vi "StopRequest.vi"(8 "error in (no error)":errorcluster, 9 "Wait for Module to stop? (F)":bool, 11 "ModuleAdmin":refnum<class "ModuleAdmin.lvclass">) -> (0 "error out":errorcluster, 2 "Stop Request Sent":bool)   [LabVIEW 2017, in "PmuImpairModule.lvlib"]
uses:
  PmuImpairModule.lvlib
  <userlib>/NIST/ModuleAdminLib/ModuleAdmin/ModuleAdmin.lvclass
  <vilib>/event_ctls.llb/usereventprio.ctl
  PublicAPI/Arguments/Requests/clStopArgument.ctl
  clEventType.ctl
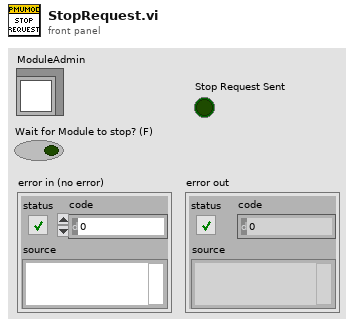
[diagram p1: front panel]
types:
  T1 = typedef "PmuImpairModule.lvlib/clRequestEvents.ctl" = cluster{"StopRequest":refnum<user-event>, "LoadPluginRequest":refnum<user-event>, "WriteImpairConfig":refnum<user-event>, "ReadImpairConfig":refnum<user-event>, "WriteImpairParams":refnum<user-event>, "ReadImpairParams":refnum<user-event>, "WriteEvtReports":refnum<user-event>, "GetImpairReports":refnum<user-event>, "ReadPathToPluginRequest":refnum<user-event>, "WriteEvtSignal":refnum<user-event>, "WriteEvtConfig":refnum<user-event>, "WriteEvtParams":refnum<user-event>, "ReadBusNumber":refnum<user-event>, "WriteBusNumber":refnum<user-event>, "ShowPanel":refnum<user-event>}
  T2 = typedef "PmuImpairModule.lvlib/clEventType.ctl" = cluster{"ModuleID":i32, "Data":variant}
  T3 = typedef "PmuImpairModule.lvlib/clStopArgument.ctl" = cluster{"Exit via Stop Module Req?":bool, "Wait for Module to stop?":bool, "ModuleAdmin":refnum<class "ModuleAdmin.lvclass">}
  T4 = typedef "usereventprio.ctl" = enum32{"high priority", "normal priority"}
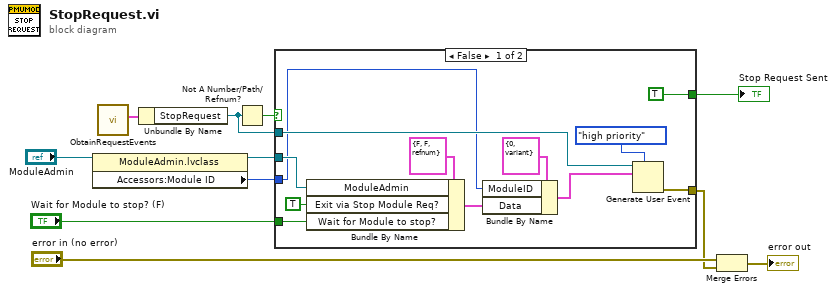
[diagram p0: block diagram]
diagram:
  n1 = property class="ModuleAdmin.lvclass"(reference="ModuleAdmin") -> (reference out=w2:refnum<class "ModuleAdmin.lvclass">, "Accessors:Module ID"=w1:i32)  [unwired: 1 in, 1 out]
  n2 = call "ObtainRequestEvents.vi"() -> ("clRequestEvents"=w11:T1)  [unwired: 10 in, 1 out]
  n3 = Unbundle By Name(w11) -> ("StopRequest"=w9:refnum<user-event>)
  n4 = Not A Number/Path/Refnum?(number/path/refnum=w9) -> (NaN/Path/Refnum?=w10:bool)
  n5 = case shown="False" w10 {
    tunnel: w9 -> [w23 _]
    tunnel: "Wait for Module to stop? (F)" -> [w16 _]
    tunnel: [w15 _] -> w5
    tunnel: [TRUE _] -> w4
    tunnel: w2 -> [w13 _]
    tunnel: w1 -> [w12 _]
    frame False {
      n6 = Bundle By Name(cluster=T3 {"Exit via Stop Module Req?"=FALSE, "Wait for Module to stop?"=FALSE, "ModuleAdmin"=refnum} ("Stop Argument"), "ModuleAdmin"=w13, "Exit via Stop Module Req?"=TRUE, "Wait for Module to stop?"=w16) -> (w18:T3)
      n7 = Bundle By Name(cluster=T2 {"ModuleID"=0, "Data"=variant} ("clBroadcast"), "ModuleID"=w12, "Data"=w18) -> (w17:T2)
      n8 = Generate User Event(priority (normal)=usereventprio."high priority", user event=w23, event data cluster=w17) -> (error out=w15:errorcluster)  [unwired: 1 in, 1 out]
    }
    frame True {
    }
  }
  "Stop Request Sent" <- w4
  n9 = Merge Errors("error in (no error)", w5) -> (→"error out":errorcluster)
